vi "Save myDLTS file (SubVI).vi"(0 "Loop data in":T10={"Persistent"={"Last file"=path "", "Last user"="", "Users"=[]}, "Temp handle"={"Connected"=FALSE, "Temp ctrl"={"Gain (P)"=0.0, "Reset (I)"=0.0, "Rate (D)"=0.0, "Stabilization rate"=0.0, "Stabilization delta"=0.0, "Type"=enum."Lake Shore 325", "Custom temp ctrl"={"VISA resource name"=""}, "Lakeshore 325"={"VISA name"="", "Loop"=0, "Heater Range"=1, "Heater Resistance"=0, "Sample sensor"=0, "Fast sensor"=0, "Slow sensor"=0}, "Lakeshore 331"={"VISA name"="", "Loop"=1, "Heater Range"=0, "Sample sensor"=0, "Fast sensor"=0, "Slow sensor"=0}, "Lakeshore 332"={"VISA name"="", "Loop"=1, "Heater Range"=0, "Sample sensor"=0, "Fast sensor"=0, "Slow sensor"=0}, "Lakeshore 335"={"VISA name"="", "Loop"=1, "Sample sensor"=0, "Fast sensor"=0, "Slow sensor"=0, "Heater Range"=0, "Output mode"=enum."Off"}, "Lakeshore 336"={"VISA name"="", "Loop"=1, "Output mode"=enum."Off", "Max current"=1.0, "Heater resistance"=1, "Sample sensor"=1, "Slow sensor"=1, "Fast sensor"=1}}}, "Paths"={"Manual"=path "", "Settings"=path "", "Persistent"=path "", "Work dir."=path ""}, "Settings"={"MFIA"={"Address"="", "Use compensation"=TRUE, "Shut down gracefully"=FALSE}, "Temp ctrl"={"Gain (P)"=0.0, "Reset (I)"=0.0, "Rate (D)"=0.0, "Stabilization rate"=0.0, "Stabilization delta"=0.0, "Type"=enum."Lake Shore 325", "Custom temp ctrl"={"VISA resource name"=""}, "Lakeshore 325"={"VISA name"="", "Loop"=0, "Heater Range"=1, "Heater Resistance"=0, "Sample sensor"=0, "Fast sensor"=0, "Slow sensor"=0}, "Lakeshore 331"={"VISA name"="", "Loop"=1, "Heater Range"=0, "Sample sensor"=0, "Fast sensor"=0, "Slow sensor"=0}, "Lakeshore 332"={"VISA name"="", "Loop"=1, "Heater Range"=0, "Sample sensor"=0, "Fast sensor"=0, "Slow sensor"=0}, "Lakeshore 335"={"VISA name"="", "Loop"=1, "Sample sensor"=0, "Fast sensor"=0, "Slow sensor"=0, "Heater Range"=0, "Output mode"=enum."Off"}, "Lakeshore 336"={"VISA name"="", "Loop"=1, "Output mode"=enum."Off", "Max current"=1.0, "Heater resistance"=1, "Sample sensor"=1, "Slow sensor"=1, "Fast sensor"=1}}, "Source-meter"={"Type"=enum."Custom", "Custom source-meter"={"VISA resource name"=""}, "Keithley 2600"={"VISA name"="", "Ignore ID Query"=FALSE, "SMU"=enum."Channel A"}, "Keithley 2400 Series"={"VISA name"="", "Ignore ID Query"=FALSE}}, "Other"={"Enable OriginLab"=FALSE, "Reader mode"=FALSE, "Auto-save"=FALSE}, "Defaults"={"IV properties"={"T"=0.0, "Vstart"=-0.5, "Vstop"=0.5, "Vpoints"=10.0, "Settling"=0.01, "I limit"=0.1, "Log mapping"=FALSE, "Averaging"=0.0}, "CV properties"={"T"=0.0, "Vstart"=-0.5, "Vstop"=0.5, "Vpoints"=10.0, "Precision"=enum."Normal", "Test signal"=0.01, "Auto I range"=FALSE, "Test frequency"=100000.0, "I range"=-2.0, "V range"=10.0, "Log mapping"=FALSE, "Rel perm"=0.0, "Area"=0.0, "Equivalent circuit model"=0}, "DLTS properties"={"Tstart"=0.0, "Instant start"=FALSE, "Tstop"=0.0, "T rate"=0.0, "Test signal"=0.0, "Test frequency"=0.0, "Bandwidth"=0.0, "Averaging"=0.0, "Vbias"=0.0, "Vpulse"=0.0, "pulse length"=0.0, "Pulse 2"=FALSE, "Vpulse 2"=0.0, "pulse length 2"=0.0, "I range"=-2.0, "V range"=10.0, "Emission rate"=[], "Sampling rate"=0.0, "Acq. delay"=0.0, "Filter order"=0, "Equivalent circuit model"=0}, "LDLTS properties"={"T"=0.0, "Test signal"=0.0, "Test frequency"=0.0, "Bandwidth"=0.0, "Averaging"=0.0, "Vbias"=0.0, "Vpulse"=0.0, "pulse length"=0.0, "Pulse 2"=FALSE, "Vpulse 2"=0.0, "pulse length 2"=0.0, "I range"=-2.0, "V range"=10.0, "Sampling rate"=0.0, "Acq. delay"=0.0, "Sampling time"=0.0, "Filter order"=0, "Equivalent circuit model"=0}}}, "Software version"=0.0, "MFIA handle"={"ziHandle"={"handleValid"=FALSE, "Conn"=0, "Path Prefix"="", "Handle"=0, "Connected"=FALSE, "Clockbase(s)"=0.0}, "Selected device"="", "ziModHandle"={"handleValid"=FALSE, "Conn"=0, "ModHandle"=0, "moduleID"="", "Path Prefix"=""}}, "Source-meter handle"={"Connected"=FALSE, "Source-meter"={"Type"=enum."Custom", "Custom source-meter"={"VISA resource name"=""}, "Keithley 2600"={"VISA name"="", "Ignore ID Query"=FALSE, "SMU"=enum."Channel A"}, "Keithley 2400 Series"={"VISA name"="", "Ignore ID Query"=FALSE}}}} {"MFIA handle"."ziModHandle"."ModHandle" format="0x%08x"; "MFIA handle"."ziModHandle"."Conn" format="0x%08x"; "MFIA handle"."ziHandle"."Handle" format="0x%08x"; "MFIA handle"."ziHandle"."Conn" format="0x%08x"; "Settings"."Defaults"."LDLTS properties"."Equivalent circuit model" items=["Rp || Cp", "Rs + Cs", "Rs + Ls", "G B", "D Cs", "Q Cs", "D Ls", "Q Ls", "Rp || Lp", "D Cp"]; "Settings"."Defaults"."LDLTS properties"."Filter order" min=0 max=8 step=1; "Settings"."Defaults"."LDLTS properties"."Sampling rate" items=["13k"=13392.857422, "27k"=26785.714844, "54k"=53571.429687, "107k"=107142.859375]; "Settings"."Defaults"."LDLTS properties"."V range" items=["10mV"=0.01, "100mV"=0.1, "1V"=1.0, "10V"=10.0]; "Settings"."Defaults"."LDLTS properties"."I range" items=["100nA"=-7.0, "1µA"=-6.0, "10µA"=-5.0, "100µA"=-4.0, "1mA"=-3.0, "10mA"=-2.0]; "Settings"."Defaults"."DLTS properties"."Equivalent circuit model" items=["Rp || Cp", "Rs + Cs", "Rs + Ls", "G B", "D Cs", "Q Cs", "D Ls", "Q Ls", "Rp || Lp", "D Cp"]; "Settings"."Defaults"."DLTS properties"."Filter order" min=0 max=8 step=1; "Settings"."Defaults"."DLTS properties"."Sampling rate" items=["13k"=13392.857422, "27k"=26785.714844, "54k"=53571.429687, "107k"=107142.859375]; "Settings"."Defaults"."DLTS properties"."V range" items=["10mV"=0.01, "100mV"=0.1, "1V"=1.0, "10V"=10.0]; "Settings"."Defaults"."DLTS properties"."I range" items=["10mV"=0.01, "100mV"=0.1, "1V"=1.0, "10V"=10.0]; "Settings"."Defaults"."CV properties"."Equivalent circuit model" items=["Rp || Cp", "Rs + Cs", "Rs + Ls", "G B", "D Cs", "Q Cs", "D Ls", "Q Ls", "Rp || Lp", "D Cp"]; "Settings"."Defaults"."CV properties"."V range" items=["10mV"=0.01, "100mV"=0.1, "1V"=1.0, "10V"=10.0]; "Settings"."Defaults"."CV properties"."I range" items=["100nA"=-7.0, "1µA"=-6.0, "10µA"=-5.0, "100µA"=-4.0, "1mA"=-3.0, "10mA"=-2.0]; "Settings"."Defaults"."IV properties"."Settling" min=0.0 max=65535.0; "Settings"."Temp ctrl"."Lakeshore 336"."Fast sensor" items=["Sensor A", "Sensor B", "Sensor C", "Sensor D"]; "Settings"."Temp ctrl"."Lakeshore 336"."Slow sensor" items=["Sensor A", "Sensor B", "Sensor C", "Sensor D"]; "Settings"."Temp ctrl"."Lakeshore 336"."Sample sensor" items=["Sensor A", "Sensor B", "Sensor C", "Sensor D"]; "Settings"."Temp ctrl"."Lakeshore 336"."Heater resistance" items=["25 Ohm"=1, "50 Ohm"=2]; "Settings"."Temp ctrl"."Lakeshore 336"."Max current" items=["0.707 A"=0.0, "1 A"=1.0, "1.414 A"=1.414, "2 A"=2.0]; "Settings"."Temp ctrl"."Lakeshore 336"."Loop" items=["Output 1"=1, "Output 2"=2, "Output 3"=3, "Output 4"=4]; "Settings"."Temp ctrl"."Lakeshore 335"."Heater Range" items=["Off", "Low (On)", "Medium", "High"]; "Settings"."Temp ctrl"."Lakeshore 335"."Slow sensor" items=["A", "B"]; "Settings"."Temp ctrl"."Lakeshore 335"."Fast sensor" items=["A", "B"]; "Settings"."Temp ctrl"."Lakeshore 335"."Sample sensor" items=["A", "B"]; "Settings"."Temp ctrl"."Lakeshore 335"."Loop" items=["Loop 1"=1, "Loop 2"=2]; "Settings"."Temp ctrl"."Lakeshore 332"."Slow sensor" items=["A", "B"]; "Settings"."Temp ctrl"."Lakeshore 332"."Fast sensor" items=["A", "B"]; "Settings"."Temp ctrl"."Lakeshore 332"."Sample sensor" items=["A", "B"]; "Settings"."Temp ctrl"."Lakeshore 332"."Heater Range" items=["Off", "Low (0.5W)", "Med (5W)", "High (50W)"]; "Settings"."Temp ctrl"."Lakeshore 332"."Loop" items=["Loop 1", "Loop 2"]; "Settings"."Temp ctrl"."Lakeshore 331"."Slow sensor" items=["A", "B"]; "Settings"."Temp ctrl"."Lakeshore 331"."Fast sensor" items=["A", "B"]; "Settings"."Temp ctrl"."Lakeshore 331"."Sample sensor" items=["A", "B"]; "Settings"."Temp ctrl"."Lakeshore 331"."Heater Range" items=["Off", "Low (0.5W)", "Med (5W)", "High (50W)"]; "Settings"."Temp ctrl"."Lakeshore 331"."Loop" items=["Loop 1", "Loop 2"]; "Settings"."Temp ctrl"."Lakeshore 325"."Slow sensor" items=["A", "B"]; "Settings"."Temp ctrl"."Lakeshore 325"."Fast sensor" items=["A", "B"]; "Settings"."Temp ctrl"."Lakeshore 325"."Sample sensor" items=["A", "B"]; "Settings"."Temp ctrl"."Lakeshore 325"."Heater Resistance" items=["25 Ohm"=1, "50 Ohm"=2]; "Settings"."Temp ctrl"."Lakeshore 325"."Heater Range" items=["Off", "Low (loop 1) or On (loop 2)", "High (loop 1)"]; "Settings"."Temp ctrl"."Lakeshore 325"."Loop" items=["Loop 1"=1, "Loop 2"=2]; "Temp handle"."Temp ctrl"."Lakeshore 336"."Fast sensor" items=["Sensor A", "Sensor B", "Sensor C", "Sensor D"]; "Temp handle"."Temp ctrl"."Lakeshore 336"."Slow sensor" items=["Sensor A", "Sensor B", "Sensor C", "Sensor D"]; "Temp handle"."Temp ctrl"."Lakeshore 336"."Sample sensor" items=["Sensor A", "Sensor B", "Sensor C", "Sensor D"]; "Temp handle"."Temp ctrl"."Lakeshore 336"."Heater resistance" items=["25 Ohm"=1, "50 Ohm"=2]; "Temp handle"."Temp ctrl"."Lakeshore 336"."Max current" items=["0.707 A"=0.0, "1 A"=1.0, "1.414 A"=1.414, "2 A"=2.0]; "Temp handle"."Temp ctrl"."Lakeshore 336"."Loop" items=["Output 1"=1, "Output 2"=2, "Output 3"=3, "Output 4"=4]; "Temp handle"."Temp ctrl"."Lakeshore 335"."Heater Range" items=["Off", "Low (On)", "Medium", "High"]; "Temp handle"."Temp ctrl"."Lakeshore 335"."Slow sensor" items=["A", "B"]; "Temp handle"."Temp ctrl"."Lakeshore 335"."Fast sensor" items=["A", "B"]; "Temp handle"."Temp ctrl"."Lakeshore 335"."Sample sensor" items=["A", "B"]; "Temp handle"."Temp ctrl"."Lakeshore 335"."Loop" items=["Loop 1"=1, "Loop 2"=2]; "Temp handle"."Temp ctrl"."Lakeshore 332"."Slow sensor" items=["A", "B"]; "Temp handle"."Temp ctrl"."Lakeshore 332"."Fast sensor" items=["A", "B"]; "Temp handle"."Temp ctrl"."Lakeshore 332"."Sample sensor" items=["A", "B"]; "Temp handle"."Temp ctrl"."Lakeshore 332"."Heater Range" items=["Off", "Low (0.5W)", "Med (5W)", "High (50W)"]; "Temp handle"."Temp ctrl"."Lakeshore 332"."Loop" items=["Loop 1", "Loop 2"]; "Temp handle"."Temp ctrl"."Lakeshore 331"."Slow sensor" items=["A", "B"]; "Temp handle"."Temp ctrl"."Lakeshore 331"."Fast sensor" items=["A", "B"]; "Temp handle"."Temp ctrl"."Lakeshore 331"."Sample sensor" items=["A", "B"]; "Temp handle"."Temp ctrl"."Lakeshore 331"."Heater Range" items=["Off", "Low (0.5W)", "Med (5W)", "High (50W)"]; "Temp handle"."Temp ctrl"."Lakeshore 331"."Loop" items=["Loop 1", "Loop 2"]; "Temp handle"."Temp ctrl"."Lakeshore 325"."Slow sensor" items=["A", "B"]; "Temp handle"."Temp ctrl"."Lakeshore 325"."Fast sensor" items=["A", "B"]; "Temp handle"."Temp ctrl"."Lakeshore 325"."Sample sensor" items=["A", "B"]; "Temp handle"."Temp ctrl"."Lakeshore 325"."Heater Resistance" items=["25 Ohm"=1, "50 Ohm"=2]; "Temp handle"."Temp ctrl"."Lakeshore 325"."Heater Range" items=["Off", "Low (loop 1) or On (loop 2)", "High (loop 1)"]; "Temp handle"."Temp ctrl"."Lakeshore 325"."Loop" items=["Loop 1"=1, "Loop 2"=2]}, 1 "Index":T1 {"IV"."IV properties"."Settling" min=0.0 max=65535.0; "CV"."CV properties"."Equivalent circuit model" items=["Rp || Cp", "Rs + Cs", "Rs + Ls", "G B", "D Cs", "Q Cs", "D Ls", "Q Ls", "Rp || Lp", "D Cp"]; "CV"."CV properties"."V range" items=["10mV"=0.01, "100mV"=0.1, "1V"=1.0, "10V"=10.0]; "CV"."CV properties"."I range" items=["100nA"=-7.0, "1µA"=-6.0, "10µA"=-5.0, "100µA"=-4.0, "1mA"=-3.0, "10mA"=-2.0]; "LDLTS"."LDLTS properties"."Equivalent circuit model" items=["Rp || Cp", "Rs + Cs", "Rs + Ls", "G B", "D Cs", "Q Cs", "D Ls", "Q Ls", "Rp || Lp", "D Cp"]; "LDLTS"."LDLTS properties"."Filter order" min=0 max=8 step=1; "LDLTS"."LDLTS properties"."Sampling rate" items=["13k"=13392.857422, "27k"=26785.714844, "54k"=53571.429687, "107k"=107142.859375]; "LDLTS"."LDLTS properties"."V range" items=["10mV"=0.01, "100mV"=0.1, "1V"=1.0, "10V"=10.0]; "LDLTS"."LDLTS properties"."I range" items=["100nA"=-7.0, "1µA"=-6.0, "10µA"=-5.0, "100µA"=-4.0, "1mA"=-3.0, "10mA"=-2.0]; "Conv DLTS"."DLTS properties"."Equivalent circuit model" items=["Rp || Cp", "Rs + Cs", "Rs + Ls", "G B", "D Cs", "Q Cs", "D Ls", "Q Ls", "Rp || Lp", "D Cp"]; "Conv DLTS"."DLTS properties"."Filter order" min=0 max=8 step=1; "Conv DLTS"."DLTS properties"."Sampling rate" items=["13k"=13392.857422, "27k"=26785.714844, "54k"=53571.429687, "107k"=107142.859375]; "Conv DLTS"."DLTS properties"."V range" items=["10mV"=0.01, "100mV"=0.1, "1V"=1.0, "10V"=10.0]; "Conv DLTS"."DLTS properties"."I range" items=["10mV"=0.01, "100mV"=0.1, "1V"=1.0, "10V"=10.0]}, 5 "Session properties":T25, 7 "Workspace path":path, 9 "File":path, 11 "Error In":errorcluster) -> (4 "Loop data out":T10={"Persistent"={"Last file"=path "", "Last user"="", "Users"=[]}, "Temp handle"={"Connected"=FALSE, "Temp ctrl"={"Gain (P)"=0.0, "Reset (I)"=0.0, "Rate (D)"=0.0, "Stabilization rate"=0.0, "Stabilization delta"=0.0, "Type"=enum."Lake Shore 325", "Custom temp ctrl"={"VISA resource name"=""}, "Lakeshore 325"={"VISA name"="", "Loop"=0, "Heater Range"=1, "Heater Resistance"=0, "Sample sensor"=0, "Fast sensor"=0, "Slow sensor"=0}, "Lakeshore 331"={"VISA name"="", "Loop"=1, "Heater Range"=0, "Sample sensor"=0, "Fast sensor"=0, "Slow sensor"=0}, "Lakeshore 332"={"VISA name"="", "Loop"=1, "Heater Range"=0, "Sample sensor"=0, "Fast sensor"=0, "Slow sensor"=0}, "Lakeshore 335"={"VISA name"="", "Loop"=1, "Sample sensor"=0, "Fast sensor"=0, "Slow sensor"=0, "Heater Range"=0, "Output mode"=enum."Off"}, "Lakeshore 336"={"VISA name"="", "Loop"=1, "Output mode"=enum."Off", "Max current"=1.0, "Heater resistance"=1, "Sample sensor"=1, "Slow sensor"=1, "Fast sensor"=1}}}, "Paths"={"Manual"=path "", "Settings"=path "", "Persistent"=path "", "Work dir."=path ""}, "Settings"={"MFIA"={"Address"="", "Use compensation"=TRUE, "Shut down gracefully"=FALSE}, "Temp ctrl"={"Gain (P)"=0.0, "Reset (I)"=0.0, "Rate (D)"=0.0, "Stabilization rate"=0.0, "Stabilization delta"=0.0, "Type"=enum."Lake Shore 325", "Custom temp ctrl"={"VISA resource name"=""}, "Lakeshore 325"={"VISA name"="", "Loop"=0, "Heater Range"=1, "Heater Resistance"=0, "Sample sensor"=0, "Fast sensor"=0, "Slow sensor"=0}, "Lakeshore 331"={"VISA name"="", "Loop"=1, "Heater Range"=0, "Sample sensor"=0, "Fast sensor"=0, "Slow sensor"=0}, "Lakeshore 332"={"VISA name"="", "Loop"=1, "Heater Range"=0, "Sample sensor"=0, "Fast sensor"=0, "Slow sensor"=0}, "Lakeshore 335"={"VISA name"="", "Loop"=1, "Sample sensor"=0, "Fast sensor"=0, "Slow sensor"=0, "Heater Range"=0, "Output mode"=enum."Off"}, "Lakeshore 336"={"VISA name"="", "Loop"=1, "Output mode"=enum."Off", "Max current"=1.0, "Heater resistance"=1, "Sample sensor"=1, "Slow sensor"=1, "Fast sensor"=1}}, "Source-meter"={"Type"=enum."Custom", "Custom source-meter"={"VISA resource name"=""}, "Keithley 2600"={"VISA name"="", "Ignore ID Query"=FALSE, "SMU"=enum."Channel A"}, "Keithley 2400 Series"={"VISA name"="", "Ignore ID Query"=FALSE}}, "Other"={"Enable OriginLab"=FALSE, "Reader mode"=FALSE, "Auto-save"=FALSE}, "Defaults"={"IV properties"={"T"=0.0, "Vstart"=-0.5, "Vstop"=0.5, "Vpoints"=10.0, "Settling"=0.01, "I limit"=0.1, "Log mapping"=FALSE, "Averaging"=0.0}, "CV properties"={"T"=0.0, "Vstart"=-0.5, "Vstop"=0.5, "Vpoints"=10.0, "Precision"=enum."Normal", "Test signal"=0.01, "Auto I range"=FALSE, "Test frequency"=100000.0, "I range"=-2.0, "V range"=10.0, "Log mapping"=FALSE, "Rel perm"=0.0, "Area"=0.0, "Equivalent circuit model"=0}, "DLTS properties"={"Tstart"=0.0, "Instant start"=FALSE, "Tstop"=0.0, "T rate"=0.0, "Test signal"=0.0, "Test frequency"=0.0, "Bandwidth"=0.0, "Averaging"=0.0, "Vbias"=0.0, "Vpulse"=0.0, "pulse length"=0.0, "Pulse 2"=FALSE, "Vpulse 2"=0.0, "pulse length 2"=0.0, "I range"=-2.0, "V range"=10.0, "Emission rate"=[], "Sampling rate"=0.0, "Acq. delay"=0.0, "Filter order"=0, "Equivalent circuit model"=0}, "LDLTS properties"={"T"=0.0, "Test signal"=0.0, "Test frequency"=0.0, "Bandwidth"=0.0, "Averaging"=0.0, "Vbias"=0.0, "Vpulse"=0.0, "pulse length"=0.0, "Pulse 2"=FALSE, "Vpulse 2"=0.0, "pulse length 2"=0.0, "I range"=-2.0, "V range"=10.0, "Sampling rate"=0.0, "Acq. delay"=0.0, "Sampling time"=0.0, "Filter order"=0, "Equivalent circuit model"=0}}}, "Software version"=0.0, "MFIA handle"={"ziHandle"={"handleValid"=FALSE, "Conn"=0, "Path Prefix"="", "Handle"=0, "Connected"=FALSE, "Clockbase(s)"=0.0}, "Selected device"="", "ziModHandle"={"handleValid"=FALSE, "Conn"=0, "ModHandle"=0, "moduleID"="", "Path Prefix"=""}}, "Source-meter handle"={"Connected"=FALSE, "Source-meter"={"Type"=enum."Custom", "Custom source-meter"={"VISA resource name"=""}, "Keithley 2600"={"VISA name"="", "Ignore ID Query"=FALSE, "SMU"=enum."Channel A"}, "Keithley 2400 Series"={"VISA name"="", "Ignore ID Query"=FALSE}}}} {"MFIA handle"."ziModHandle"."ModHandle" format="0x%08x"; "MFIA handle"."ziModHandle"."Conn" format="0x%08x"; "MFIA handle"."ziHandle"."Handle" format="0x%08x"; "MFIA handle"."ziHandle"."Conn" format="0x%08x"; "Settings"."Defaults"."LDLTS properties"."Equivalent circuit model" items=["Rp || Cp", "Rs + Cs", "Rs + Ls", "G B", "D Cs", "Q Cs", "D Ls", "Q Ls", "Rp || Lp", "D Cp"]; "Settings"."Defaults"."LDLTS properties"."Filter order" min=0 max=8 step=1; "Settings"."Defaults"."LDLTS properties"."Sampling rate" items=["13k"=13392.857422, "27k"=26785.714844, "54k"=53571.429687, "107k"=107142.859375]; "Settings"."Defaults"."LDLTS properties"."V range" items=["10mV"=0.01, "100mV"=0.1, "1V"=1.0, "10V"=10.0]; "Settings"."Defaults"."LDLTS properties"."I range" items=["100nA"=-7.0, "1µA"=-6.0, "10µA"=-5.0, "100µA"=-4.0, "1mA"=-3.0, "10mA"=-2.0]; "Settings"."Defaults"."DLTS properties"."Equivalent circuit model" items=["Rp || Cp", "Rs + Cs", "Rs + Ls", "G B", "D Cs", "Q Cs", "D Ls", "Q Ls", "Rp || Lp", "D Cp"]; "Settings"."Defaults"."DLTS properties"."Filter order" min=0 max=8 step=1; "Settings"."Defaults"."DLTS properties"."Sampling rate" items=["13k"=13392.857422, "27k"=26785.714844, "54k"=53571.429687, "107k"=107142.859375]; "Settings"."Defaults"."DLTS properties"."V range" items=["10mV"=0.01, "100mV"=0.1, "1V"=1.0, "10V"=10.0]; "Settings"."Defaults"."DLTS properties"."I range" items=["10mV"=0.01, "100mV"=0.1, "1V"=1.0, "10V"=10.0]; "Settings"."Defaults"."CV properties"."Equivalent circuit model" items=["Rp || Cp", "Rs + Cs", "Rs + Ls", "G B", "D Cs", "Q Cs", "D Ls", "Q Ls", "Rp || Lp", "D Cp"]; "Settings"."Defaults"."CV properties"."V range" items=["10mV"=0.01, "100mV"=0.1, "1V"=1.0, "10V"=10.0]; "Settings"."Defaults"."CV properties"."I range" items=["100nA"=-7.0, "1µA"=-6.0, "10µA"=-5.0, "100µA"=-4.0, "1mA"=-3.0, "10mA"=-2.0]; "Settings"."Defaults"."IV properties"."Settling" min=0.0 max=65535.0; "Settings"."Temp ctrl"."Lakeshore 336"."Fast sensor" items=["Sensor A", "Sensor B", "Sensor C", "Sensor D"]; "Settings"."Temp ctrl"."Lakeshore 336"."Slow sensor" items=["Sensor A", "Sensor B", "Sensor C", "Sensor D"]; "Settings"."Temp ctrl"."Lakeshore 336"."Sample sensor" items=["Sensor A", "Sensor B", "Sensor C", "Sensor D"]; "Settings"."Temp ctrl"."Lakeshore 336"."Heater resistance" items=["25 Ohm"=1, "50 Ohm"=2]; "Settings"."Temp ctrl"."Lakeshore 336"."Max current" items=["0.707 A"=0.0, "1 A"=1.0, "1.414 A"=1.414, "2 A"=2.0]; "Settings"."Temp ctrl"."Lakeshore 336"."Loop" items=["Output 1"=1, "Output 2"=2, "Output 3"=3, "Output 4"=4]; "Settings"."Temp ctrl"."Lakeshore 335"."Heater Range" items=["Off", "Low (On)", "Medium", "High"]; "Settings"."Temp ctrl"."Lakeshore 335"."Slow sensor" items=["A", "B"]; "Settings"."Temp ctrl"."Lakeshore 335"."Fast sensor" items=["A", "B"]; "Settings"."Temp ctrl"."Lakeshore 335"."Sample sensor" items=["A", "B"]; "Settings"."Temp ctrl"."Lakeshore 335"."Loop" items=["Loop 1"=1, "Loop 2"=2]; "Settings"."Temp ctrl"."Lakeshore 332"."Slow sensor" items=["A", "B"]; "Settings"."Temp ctrl"."Lakeshore 332"."Fast sensor" items=["A", "B"]; "Settings"."Temp ctrl"."Lakeshore 332"."Sample sensor" items=["A", "B"]; "Settings"."Temp ctrl"."Lakeshore 332"."Heater Range" items=["Off", "Low (0.5W)", "Med (5W)", "High (50W)"]; "Settings"."Temp ctrl"."Lakeshore 332"."Loop" items=["Loop 1", "Loop 2"]; "Settings"."Temp ctrl"."Lakeshore 331"."Slow sensor" items=["A", "B"]; "Settings"."Temp ctrl"."Lakeshore 331"."Fast sensor" items=["A", "B"]; "Settings"."Temp ctrl"."Lakeshore 331"."Sample sensor" items=["A", "B"]; "Settings"."Temp ctrl"."Lakeshore 331"."Heater Range" items=["Off", "Low (0.5W)", "Med (5W)", "High (50W)"]; "Settings"."Temp ctrl"."Lakeshore 331"."Loop" items=["Loop 1", "Loop 2"]; "Settings"."Temp ctrl"."Lakeshore 325"."Slow sensor" items=["A", "B"]; "Settings"."Temp ctrl"."Lakeshore 325"."Fast sensor" items=["A", "B"]; "Settings"."Temp ctrl"."Lakeshore 325"."Sample sensor" items=["A", "B"]; "Settings"."Temp ctrl"."Lakeshore 325"."Heater Resistance" items=["25 Ohm"=1, "50 Ohm"=2]; "Settings"."Temp ctrl"."Lakeshore 325"."Heater Range" items=["Off", "Low (loop 1) or On (loop 2)", "High (loop 1)"]; "Settings"."Temp ctrl"."Lakeshore 325"."Loop" items=["Loop 1"=1, "Loop 2"=2]; "Temp handle"."Temp ctrl"."Lakeshore 336"."Fast sensor" items=["Sensor A", "Sensor B", "Sensor C", "Sensor D"]; "Temp handle"."Temp ctrl"."Lakeshore 336"."Slow sensor" items=["Sensor A", "Sensor B", "Sensor C", "Sensor D"]; "Temp handle"."Temp ctrl"."Lakeshore 336"."Sample sensor" items=["Sensor A", "Sensor B", "Sensor C", "Sensor D"]; "Temp handle"."Temp ctrl"."Lakeshore 336"."Heater resistance" items=["25 Ohm"=1, "50 Ohm"=2]; "Temp handle"."Temp ctrl"."Lakeshore 336"."Max current" items=["0.707 A"=0.0, "1 A"=1.0, "1.414 A"=1.414, "2 A"=2.0]; "Temp handle"."Temp ctrl"."Lakeshore 336"."Loop" items=["Output 1"=1, "Output 2"=2, "Output 3"=3, "Output 4"=4]; "Temp handle"."Temp ctrl"."Lakeshore 335"."Heater Range" items=["Off", "Low (On)", "Medium", "High"]; "Temp handle"."Temp ctrl"."Lakeshore 335"."Slow sensor" items=["A", "B"]; "Temp handle"."Temp ctrl"."Lakeshore 335"."Fast sensor" items=["A", "B"]; "Temp handle"."Temp ctrl"."Lakeshore 335"."Sample sensor" items=["A", "B"]; "Temp handle"."Temp ctrl"."Lakeshore 335"."Loop" items=["Loop 1"=1, "Loop 2"=2]; "Temp handle"."Temp ctrl"."Lakeshore 332"."Slow sensor" items=["A", "B"]; "Temp handle"."Temp ctrl"."Lakeshore 332"."Fast sensor" items=["A", "B"]; "Temp handle"."Temp ctrl"."Lakeshore 332"."Sample sensor" items=["A", "B"]; "Temp handle"."Temp ctrl"."Lakeshore 332"."Heater Range" items=["Off", "Low (0.5W)", "Med (5W)", "High (50W)"]; "Temp handle"."Temp ctrl"."Lakeshore 332"."Loop" items=["Loop 1", "Loop 2"]; "Temp handle"."Temp ctrl"."Lakeshore 331"."Slow sensor" items=["A", "B"]; "Temp handle"."Temp ctrl"."Lakeshore 331"."Fast sensor" items=["A", "B"]; "Temp handle"."Temp ctrl"."Lakeshore 331"."Sample sensor" items=["A", "B"]; "Temp handle"."Temp ctrl"."Lakeshore 331"."Heater Range" items=["Off", "Low (0.5W)", "Med (5W)", "High (50W)"]; "Temp handle"."Temp ctrl"."Lakeshore 331"."Loop" items=["Loop 1", "Loop 2"]; "Temp handle"."Temp ctrl"."Lakeshore 325"."Slow sensor" items=["A", "B"]; "Temp handle"."Temp ctrl"."Lakeshore 325"."Fast sensor" items=["A", "B"]; "Temp handle"."Temp ctrl"."Lakeshore 325"."Sample sensor" items=["A", "B"]; "Temp handle"."Temp ctrl"."Lakeshore 325"."Heater Resistance" items=["25 Ohm"=1, "50 Ohm"=2]; "Temp handle"."Temp ctrl"."Lakeshore 325"."Heater Range" items=["Off", "Low (loop 1) or On (loop 2)", "High (loop 1)"]; "Temp handle"."Temp ctrl"."Lakeshore 325"."Loop" items=["Loop 1"=1, "Loop 2"=2]}, 6 "Session properties out":T25, 8 "Workspace out":path, 10 "File path out":path, 15 "Error  out":errorcluster)   [LabVIEW 2019]
doc: "Saves session file from workspace to original location, displays a progress bar"
uses:
  <vilib>/Utility/miscctls.llb/LVPointTypeDef.ctl
  064cd131-08d2-4421-abd1-8a9001b0b0a7.vi
  Type defs/Temp handle Type Def.ctl
  Type defs/Persistent Type Def.ctl
  <instrlib>/Zurich Instruments LabOne/Public/ziTypeHandle.ctl
  <instrlib>/Zurich Instruments LabOne/Zurich Instruments LabOne.lvlib
  Type defs/Paths Type Def.ctl
  Type defs/Imps Type Def.ctl
  Type defs/Temp ctrl Type Def.ctl
  Type defs/Other settings Type Def.ctl
  Type defs/Settings Type Def.ctl
  Type defs/Loop data Type Def.ctl
  Type defs/Session properties Type Def.ctl
  Type defs/MFIA handle Type Def.ctl
  Type defs/DLTS properties Type Def.ctl
  Type defs/LDLTS properties Type Def.ctl
  Type defs/CV properties Type Def.ctl
  Type defs/IV properties Type Def.ctl
  Type defs/Session internal index Type Def.ctl
  Type defs/CV measurement Type Def.ctl
  Type defs/IV measurement Type Def.ctl
  <instrlib>/Zurich Instruments LabOne/Public/Modules/ziTypeModHandle.ctl
  Type defs/cDLTS measurement Type Def.ctl
  Type defs/LDLTS measurement Type Def.ctl
  Type defs/Source-meter Type Def.ctl
  Custom devices/Custom temp ctrl settings.ctl
  Custom devices/Custom source-meter settings.ctl
  Type defs/Source-meter handle Type Def.ctl
panel:
  out "Animated picture":u16(ring)
  out "String":string
  out "Progress":u8(slide) max=4 scale=0.0..5.0
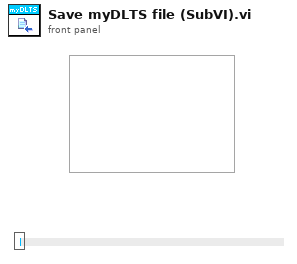
[diagram p1: front panel]
types:
  T1 = typedef "Session internal index Type Def.ctl" = cluster{"IV":T2[], "CV":T4[], "LDLTS":T6[], "Conv DLTS":T8[]}
  T2 = typedef "IV measurement Type Def.ctl" = cluster{"Name":string, "Comment":string, "Time":timestamp, "Folder":path, "IV properties":T3, "GUID":string}
  T3 = typedef "IV properties Type Def.ctl" = cluster{"T":dbl[unit], "Vstart":dbl[unit], "Vstop":dbl[unit], "Vpoints":dbl, "Settling":dbl[unit], "I limit":dbl[unit], "Log mapping":bool, "Averaging":dbl}
  T4 = typedef "CV measurement Type Def.ctl" = cluster{"Name":string, "Comment":string, "Time":timestamp, "Folder":path, "CV properties":T5, "GUID":string}
  T5 = typedef "CV properties Type Def.ctl" = cluster{"T":dbl[unit], "Vstart":dbl[unit], "Vstop":dbl[unit], "Vpoints":dbl, "Precision":enum16{"Low (Fast)", "Normal", "High (Slow)"}, "Test signal":dbl[unit], "Auto I range":bool, "Test frequency":dbl[unit], "I range":dbl, "V range":dbl[unit], "Log mapping":bool, "Rel perm":dbl, "Area":dbl[unit], "Equivalent circuit model":u16}
  T6 = typedef "LDLTS measurement Type Def.ctl" = cluster{"Name":string, "Comment":string, "Time":timestamp, "Folder":path, "LDLTS properties":T7, "GUID":string}
  T7 = typedef "LDLTS properties Type Def.ctl" = cluster{"T":dbl[unit], "Test signal":dbl[unit], "Test frequency":dbl[unit], "Bandwidth":dbl[unit], "Averaging":dbl, "Vbias":dbl[unit], "Vpulse":dbl[unit], "pulse length":dbl[unit], "Pulse 2":bool, "Vpulse 2":dbl[unit], "pulse length 2":dbl[unit], "I range":dbl, "V range":dbl[unit], "Sampling rate":dbl[unit], "Acq. delay":dbl[unit], "Sampling time":dbl[unit], "Filter order":i32, "Equivalent circuit model":u16}
  T8 = typedef "cDLTS measurement Type Def.ctl" = cluster{"Name":string, "Comment":string, "Time":timestamp, "Folder":path, "DLTS properties":T9, "GUID":string}
  T9 = typedef "DLTS properties Type Def.ctl" = cluster{"Tstart":dbl[unit], "Instant start":bool, "Tstop":dbl[unit], "T rate":dbl[unit], "Test signal":dbl[unit], "Test frequency":dbl[unit], "Bandwidth":dbl[unit], "Averaging":dbl, "Vbias":dbl[unit], "Vpulse":dbl[unit], "pulse length":dbl[unit], "Pulse 2":bool, "Vpulse 2":dbl[unit], "pulse length 2":dbl[unit], "I range":dbl, "V range":dbl[unit], "Emission rate":dbl[unit][], "Sampling rate":dbl[unit], "Acq. delay":dbl[unit], "Filter order":i32, "Equivalent circuit model":u16}
  T10 = typedef "Loop data Type Def.ctl" = cluster{"Persistent":T11, "Temp handle":T12, "Paths":T15, "Settings":T16, "Software version":dbl, "MFIA handle":T21, "Source-meter handle":T24}
  T11 = typedef "Persistent Type Def.ctl" = cluster{"Last file":path, "Last user":string, "Users":cluster{"User":string, "Authors directory":path}[]}
  T12 = typedef "Temp handle Type Def.ctl" = cluster{"Connected":bool, "Temp ctrl":T13}
  T13 = typedef "Temp ctrl Type Def.ctl" = cluster{"Gain (P)":dbl, "Reset (I)":dbl, "Rate (D)":dbl, "Stabilization rate":dbl, "Stabilization delta":dbl, "Type":enum16{"Custom", "Lake Shore 325", "Lake Shore 331", "Lake Shore 332", "Lake Shore 335", "Lake Shore 336"}, "Custom temp ctrl":T14, "Lakeshore 325":cluster{"VISA name":refnum<visa-resource-name>, "Loop":u16, "Heater Range":u16, "Heater Resistance":u16, "Sample sensor":u16, "Fast sensor":u16, "Slow sensor":u16}, "Lakeshore 331":cluster{"VISA name":refnum<visa-resource-name>, "Loop":u16, "Heater Range":u16, "Sample sensor":u16, "Fast sensor":u16, "Slow sensor":u16}, "Lakeshore 332":cluster{"VISA name":refnum<visa-resource-name>, "Loop":u16, "Heater Range":u16, "Sample sensor":u16, "Fast sensor":u16, "Slow sensor":u16}, "Lakeshore 335":cluster{"VISA name":refnum<visa-resource-name>, "Loop":u16, "Sample sensor":u16, "Fast sensor":u16, "Slow sensor":u16, "Heater Range":u16, "Output mode":enum16{"Off", "Closed Loop PID", "Zone", "Open Loop", "Monitor Out", "Warmup Supply"}}, "Lakeshore 336":cluster{"VISA name":refnum<visa-resource-name>, "Loop":u16, "Output mode":enum16{"Off", "Closed Loop PID", "Zone", "Open Loop"}, "Max current":dbl, "Heater resistance":u16, "Sample sensor":u16, "Slow sensor":u16, "Fast sensor":u16}}
  T14 = typedef "Custom temp ctrl settings.ctl" = cluster{"VISA resource name":refnum<visa-resource-name>}
  T15 = typedef "Paths Type Def.ctl" = cluster{"Manual":path, "Settings":path, "Persistent":path, "Work dir.":path}
  T16 = typedef "Settings Type Def.ctl" = cluster{"MFIA":T17, "Temp ctrl":T13, "Source-meter":T18, "Other":T20, "Defaults":cluster{"IV properties":T3, "CV properties":T5, "DLTS properties":T9, "LDLTS properties":T7}}
  T17 = typedef "Imps Type Def.ctl" = cluster{"Address":string, "Use compensation":bool, "Shut down gracefully":bool}
  T18 = typedef "Source-meter Type Def.ctl" = cluster{"Type":enum16{"Custom", "Keithley 2600", "Keithley 2400 Series"}, "Custom source-meter":T19, "Keithley 2600":cluster{"VISA name":refnum<visa-resource-name>, "Ignore ID Query":bool, "SMU":enum16{"Channel A", "Channel B"}}, "Keithley 2400 Series":cluster{"VISA name":refnum<visa-resource-name>, "Ignore ID Query":bool}}
  T19 = typedef "Custom source-meter settings.ctl" = cluster{"VISA resource name":refnum<visa-resource-name>}
  T20 = typedef "Other settings Type Def.ctl" = cluster{"Enable OriginLab":bool, "Reader mode":bool, "Auto-save":bool}
  T21 = typedef "MFIA handle Type Def.ctl" = cluster{"ziHandle":T22, "Selected device":string, "ziModHandle":T23}
  T22 = typedef "Zurich Instruments LabOne.lvlib/ziTypeHandle.ctl" = cluster{"handleValid":bool, "Conn":u64, "Path Prefix":string, "Handle":u64, "Connected":bool, "Clockbase(s)":dbl}
  T23 = typedef "Zurich Instruments LabOne.lvlib/ziTypeModHandle.ctl" = cluster{"handleValid":bool, "Conn":u64, "ModHandle":u64, "moduleID":string, "Path Prefix":string}
  T24 = typedef "Source-meter handle Type Def.ctl" = cluster{"Connected":bool, "Source-meter":T18}
  T25 = typedef "Session properties Type Def.ctl" = cluster{"Session name":string, "Comment":string, "User":string, "Software version":dbl, "Created":timestamp, "Modified":timestamp, "Binary":bool, "GUID":string}
  T26 = typedef "LVPointTypeDef.ctl" = cluster{"Horizontal":i16, "Vertical":i16}
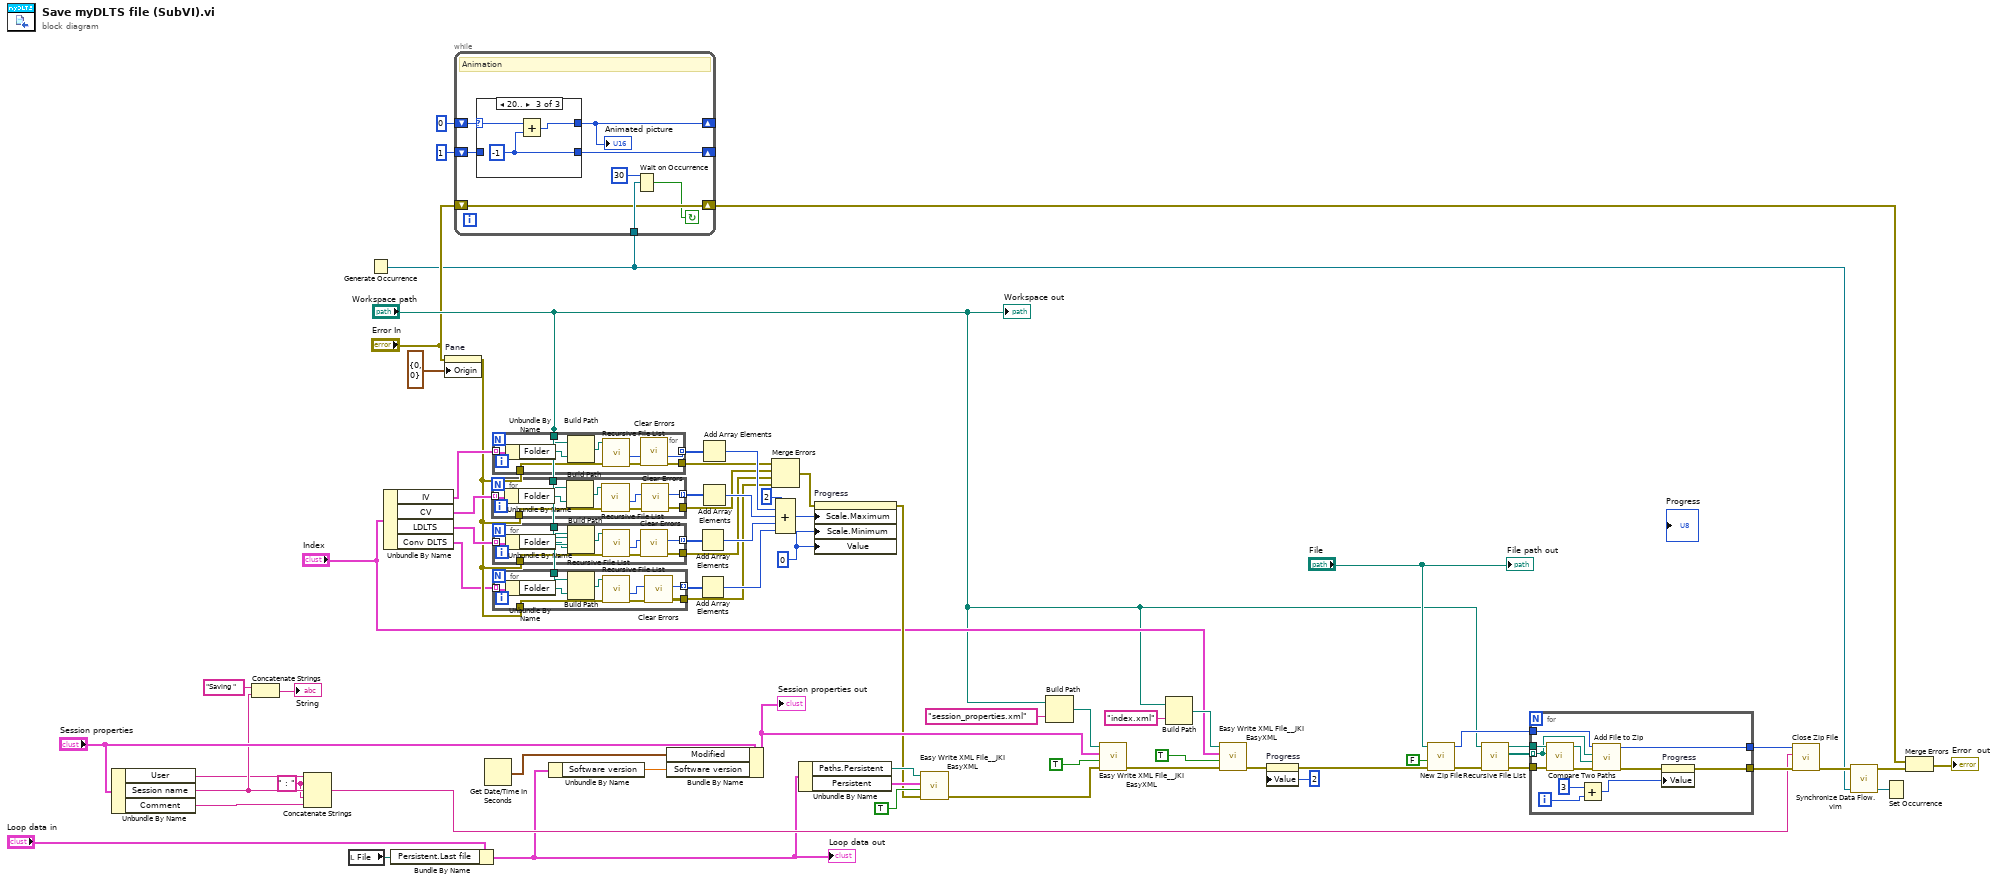
[diagram p0: block diagram]
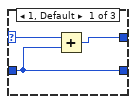
[diagram p2: hidden frame]
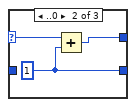
[diagram p3: hidden frame]
diagram:
  w23 = " : " ("string")
  w58 = u8 0 ("Progress")
  n1 = Unbundle By Name("Session properties") -> ("User"=w24:string, "Session name"=w27:string, "Comment"=w26:string)
  n2 = Concatenate Strings("Saving " ("string"), w27) -> (→"String":string)
  n3 = Concatenate Strings(w24, w23, w27, w23, w26) -> (w25:string)
  n4 = local read "File"() -> (w54:path)
  n5 = Generate Occurrence() -> (w2:refnum<k4>)
  n6 = Unbundle By Name("Index") -> ("IV"=w51:T2[], "CV"=w22:T4[], "LDLTS"=w17:T6[], "Conv DLTS"=w13:T8[])
  n7 = Bundle By Name(cluster="Loop data in", "Persistent.Last file"=w54) -> (w11:T10)
  "Loop data out" <- w11
  n8 = property on="Pane" class="Pane"(error in="Error In", "Origin"=T26 {"Horizontal"=0, "Vertical"=0}) -> (error out=w16:errorcluster)  [unwired: 1 in, 1 out]
  n9 = while {
    shift-right: [w78] -> _
    shift-left: u16 0 -> [w79]
    shift-right: [w76] -> _
    shift-left: i16 1 ("y") -> [w77]
    shift-right: [w74] -> w5
    shift-left: "Error In" -> [w74]
    tunnel: w2 -> [w75]
    stop <- w72 continue-if-true
    # "Animation"
    n10 = case shown="20.." w79 {
      selector: w79 -> [w82 w85 w88]
      tunnel: [w81 w84 w87] -> w78
      tunnel: w77 -> [w80 _ _]
      tunnel: [w80 w83 w86] -> w76
      frame 1, Default {
        n11 = Add(x=w82, y=w80) -> (x+y=w81:u16)
      }
      frame ..0 {
        w83 = i16 1 ("y")
        n12 = Add(x=w85, y=w83) -> (x+y=w84:u16)
      }
      frame 20.. {
        w86 = i16 -1 ("y")
        n13 = Add(x=w88, y=w86) -> (x+y=w87:u16)
      }
    }
    "Animated picture" <- w78
    n14 = Wait on Occurrence(2:w75, 3:u32 30 ("milliseconds to wait")) -> (0:w72:bool)  [unwired: 1 in]
  }
  n15 = Get Date/Time In Seconds() -> (seconds since 1Jan1904=w70:timestamp)
  n16 = for {
    tunnel: w22 -> [w96] mode=indexing
    tunnel: [w95] -> w21 mode=indexing
    tunnel: w16 -> [w94]
    tunnel: [w90] -> w20
    tunnel: "Workspace path" -> [w91]
    n17 = Unbundle By Name(w96) -> ("Folder"=w93:path)
    n18 = Build Path(base path=w91, name or relative path=w93) -> (appended path=w92:path)
    n19 = call <vilib>:"Recursive File List.vi"("error in (no error)"=w94, "Folder Path"=w92) -> ("error out"=w89:errorcluster, "Number of Files"=w95:i32)  [unwired: 5 in, 3 out]
    n20 = call <vilib>:"Clear Errors.vi"("error in (no error)"=w89) -> ("error out"=w90:errorcluster)  [unwired: 5 in, 1 out]
  }
  n21 = for {
    tunnel: w51 -> [w104] mode=indexing
    tunnel: [w103] -> w52 mode=indexing
    tunnel: w16 -> [w102]
    tunnel: [w97] -> w37
    tunnel: "Workspace path" -> [w99]
    n22 = Unbundle By Name(w104) -> ("Folder"=w101:path)
    n23 = Build Path(base path=w99, name or relative path=w101) -> (appended path=w100:path)
    n24 = call <vilib>:"Recursive File List.vi"("error in (no error)"=w102, "Folder Path"=w100) -> ("error out"=w98:errorcluster, "Number of Files"=w103:i32)  [unwired: 5 in, 3 out]
    n25 = call <vilib>:"Clear Errors.vi"("error in (no error)"=w98) -> ("error out"=w97:errorcluster)  [unwired: 5 in, 1 out]
  }
  n26 = for {
    tunnel: w17 -> [w112] mode=indexing
    tunnel: [w111] -> w18 mode=indexing
    tunnel: w16 -> [w110]
    tunnel: [w105] -> w19
    tunnel: "Workspace path" -> [w107]
    n27 = Unbundle By Name(w112) -> ("Folder"=w109:path)
    n28 = Build Path(base path=w107, name or relative path=w109) -> (appended path=w108:path)
    n29 = call <vilib>:"Recursive File List.vi"("error in (no error)"=w110, "Folder Path"=w108) -> ("error out"=w106:errorcluster, "Number of Files"=w111:i32)  [unwired: 5 in, 3 out]
    n30 = call <vilib>:"Clear Errors.vi"("error in (no error)"=w106) -> ("error out"=w105:errorcluster)  [unwired: 5 in, 1 out]
  }
  n31 = for {
    tunnel: w13 -> [w120] mode=indexing
    tunnel: [w119] -> w15 mode=indexing
    tunnel: w16 -> [w118]
    tunnel: [w113] -> w14
    tunnel: "Workspace path" -> [w115]
    n32 = Unbundle By Name(w120) -> ("Folder"=w117:path)
    n33 = Build Path(base path=w115, name or relative path=w117) -> (appended path=w116:path)
    n34 = call <vilib>:"Recursive File List.vi"("error in (no error)"=w118, "Folder Path"=w116) -> ("error out"=w114:errorcluster, "Number of Files"=w119:i32)  [unwired: 5 in, 3 out]
    n35 = call <vilib>:"Clear Errors.vi"("error in (no error)"=w114) -> ("error out"=w113:errorcluster)  [unwired: 5 in, 1 out]
  }
  n36 = Unbundle By Name(w11) -> ("Software version"=w10:dbl)
  n37 = Bundle By Name(cluster="Session properties", "Modified"=w70, "Software version"=w10) -> (w43:T25)
  "Session properties out" <- w43
  n38 = Add Array Elements(numeric array=w18) -> (sum=w49:i32)
  n39 = Add Array Elements(numeric array=w15) -> (sum=w50:i32)
  n40 = Add Array Elements(numeric array=w52) -> (sum=w47:i32)
  n41 = Add Array Elements(numeric array=w21) -> (sum=w48:i32)
  n42 = Merge Errors(w37, w20, w19, w14) -> (w36:errorcluster)
  n43 = Compound Arithmetic op=ADD(2 ("value"), w47, w48, w49, w50) -> (w60:i32)
  n44 = Unbundle By Name(w11) -> ("Paths.Persistent"=w64:path, "Persistent"=w65:T11)
  n45 = property on="Progress" class="Slide (strict)"(error in=w36, "Scale.Maximum"=w60, "Scale.Minimum"=w58, "Value"=w58) -> (error out=w41:errorcluster)  [unwired: 1 in, 1 out]
  n46 = call <vilib>:"Easy Write XML File__JKI EasyXML.vi"("error in (no error)"=w41, "Overwrite File? (false)"=TRUE, "LabVIEW Data"=w65, "XML File Path"=w64) -> ("error out"=w42:errorcluster)  [unwired: 6 in, 1 out]
  n47 = Build Path(base path="Workspace path", name or relative path="session_properties.xml") -> (appended path=w69:path)
  n48 = call <vilib>:"Easy Write XML File__JKI EasyXML.vi"("error in (no error)"=w42, "Overwrite File? (false)"=TRUE, "LabVIEW Data"=w43, "XML File Path"=w69) -> ("error out"=w40:errorcluster)  [unwired: 6 in, 1 out]
  n49 = Build Path(base path="Workspace path", name or relative path="index.xml") -> (appended path=w46:path)
  n50 = call <vilib>:"Easy Write XML File__JKI EasyXML.vi"("error in (no error)"=w40, "Overwrite File? (false)"=TRUE, "LabVIEW Data"="Index", "XML File Path"=w46) -> ("error out"=w39:errorcluster)  [unwired: 6 in, 1 out]
  n51 = property on="Progress" class="Slide (strict)"(error in=w39, "Value"=u8 2 ("Horizontal Progress Bar")) -> (error out=w59:errorcluster)  [unwired: 1 in, 1 out]
  n52 = call <vilib>:"New Zip File.vi"("error in (no error)"=w59, "confirm overwrite? (F)"=FALSE, "target"="File") -> ("error out"=w32:errorcluster, "zip file out"=w31:i64)  [unwired: 2 in, 1 out]
  n53 = call <vilib>:"Recursive File List.vi"("error in (no error)"=w32, "Folder Path"="Workspace path") -> ("error out"=w33:errorcluster, "All Files in Dir"=w35:path[], "dup Folder Path"=w34:path)  [unwired: 5 in, 2 out]
  n54 = for {
    tunnel: w35 -> [w127] mode=indexing
    tunnel: w34 -> [w131]
    tunnel: w33 -> [w132]
    tunnel: [w123] -> w30
    tunnel: [w122] -> w29
    tunnel: w31 -> [w121]
    i -> [w126]
    n55 = call <vilib>:"Compare Two Paths.vi"("error in (no error)"=w132, "Path 2"=w127, "Path 1"=w131) -> ("error out"=w129:errorcluster, "Relative Path from 1 to 2"=w128:path)  [unwired: 5 in, 2 out]
    n56 = Add(x=3, y=w126) -> (x+y=w124:i32)
    n57 = call <vilib>:"Add File to Zip.vi"("error in (no error)"=w129, "destination path in zip"=w128, "source file path"=w127, "zip file in"=w121) -> ("error out"=w130:errorcluster, "zip file out"=w122:i64)  [unwired: 6 in]
    n58 = property on="Progress" class="Slide (strict)"(error in=w130, "Value"=w124) -> (error out=w123:errorcluster)  [unwired: 1 in, 1 out]
  }
  n59 = call <vilib>:"Close Zip File.vi"("error in (no error)"=w30, "comments"=w25, "zip file in"=w29) -> ("error out"=w4:errorcluster)  [unwired: 4 in]
  n60 = call "Synchronize Data Flow.vim"("input 4"=w2, "input 1"=w4) -> ("output 4"=w1:refnum<k4>, "output 1"=w3:errorcluster)  [unwired: 2 in, 2 out]
  n61 = Set Occurrence(w1) -> ()
  n62 = Merge Errors(w5, w3) -> (→"Error  out":errorcluster)
  "File path out" <- "File"
  "Workspace out" <- "Workspace path"
